vi "Set Framed Project Path.vi"(8 "error in (no error)":errorcluster, 10 "Framed Project Path":path, 11 "Project Model in":refnum<class "Project Model.lvclass">) -> (0 "error out":errorcluster, 3 "Project Model out":refnum<class "Project Model.lvclass">)   [LabVIEW 2013, in "Project Model.lvlib" / "Project Model.lvclass"]
uses:
  Project Model.lvclass
  Project Model.lvclass/Project Model.ctl
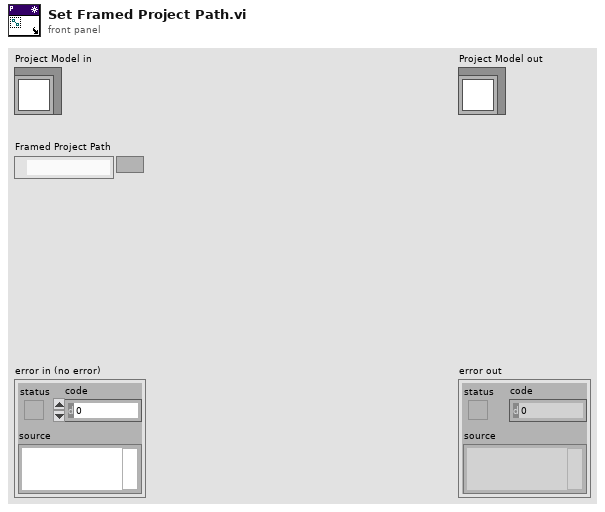
[diagram p1: front panel]
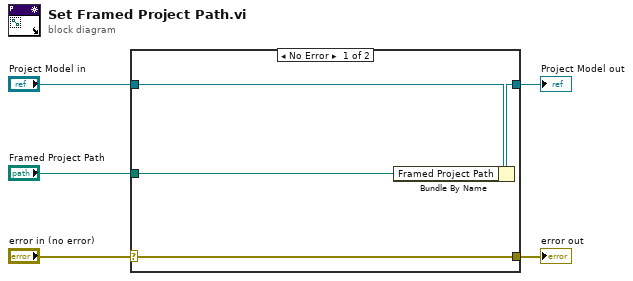
[diagram p0: block diagram]
diagram:
  n1 = case shown="No Error" "error in (no error)" {
    selector: "error in (no error)" -> [w9 w10]
    tunnel: [w9 w10] -> w4
    tunnel: [w7 w11] -> w2
    tunnel: "Project Model in" -> [w8 w11]
    tunnel: "Framed Project Path" -> [w6 _]
    frame No Error {
      n2 = Bundle By Name(cluster=w8, "Framed Project Path"=w6) -> (w7:refnum<class "Project Model.lvclass">)
    }
    frame Error {
    }
  }
  "error out" <- w4
  "Project Model out" <- w2
